vi "addNullElement.vi"(7 "Name":string, 8 "error in (no error)":errorcluster, 10 "Replace? (false)":bool, 11 "tBSONDocument in":refnum<class "tBSONDocument.lvclass">) -> (0 "error out":errorcluster, 3 "tBSONDocument out":refnum<class "tBSONDocument.lvclass">)   [LabVIEW 2013, in "BSON.lvlib" / "tBSONDocument.lvclass"]
doc: "Adds an Null element to a BSON document."
uses:
  tBSONDocument.lvclass
  BSONElements/tBSONNull/tBSONNull.lvclass
  tBSONElement/tBSONElement.lvclass
  tBSONElement/setName.vi
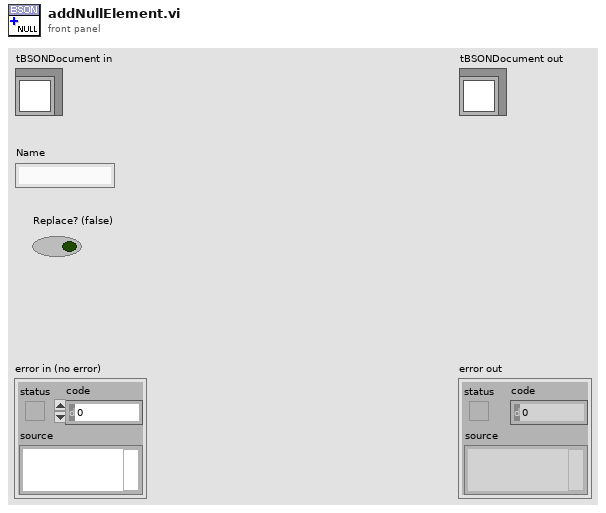
[diagram p1: front panel]
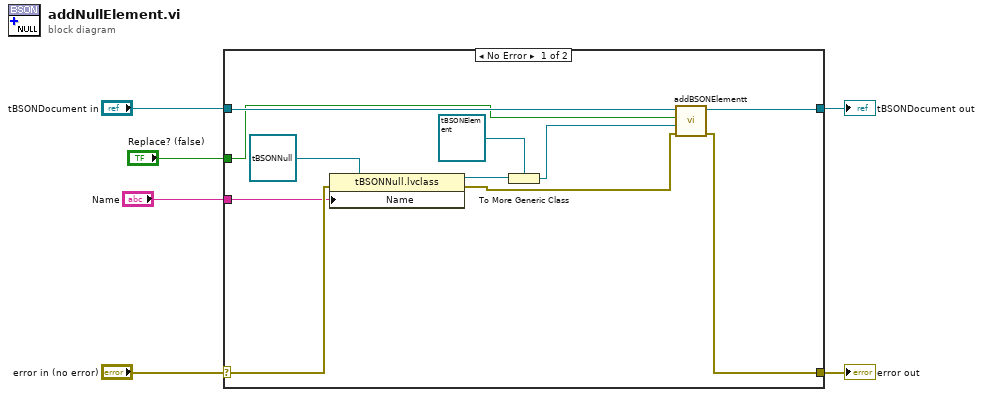
[diagram p0: block diagram]
diagram:
  n1 = case shown="No Error" "error in (no error)" {
    selector: "error in (no error)" -> [w16 w19]
    tunnel: [w9 w19] -> w5
    tunnel: [w8 w18] -> w3
    tunnel: "tBSONDocument in" -> [w14 w18]
    tunnel: "Name" -> [w15 _]
    tunnel: "Replace? (false)" -> [w7 _]
    frame No Error {
      n2 = property class="tBSONNull.lvclass"(reference=refnum<class "tBSONNull.lvclass"> refnum ("BSON.lvlib:tBSONNull.lvclass"), error in=w16, "Name"=w15) -> (reference out=w13:refnum<class "tBSONNull.lvclass">, error out=w10:errorcluster)
      n3 = To More Generic Class(target class=refnum<class "tBSONElement.lvclass"> refnum ("BSON.lvlib:tBSONElement.lvclass"), reference=w13) -> (generic class reference=w11:refnum<class "tBSONElement.lvclass">)
      n4 = call "addBSONElementt.vi"("error in (no error)"=w10, "Element"=w11, "Replace? (false)"=w7, "tBSONDocument in"=w14) -> ("error out"=w9:errorcluster, "tBSONDocument out"=w8:refnum<class "tBSONDocument.lvclass">)  [unwired: 6 in]
    }
    frame Error {
    }
  }
  "error out" <- w5
  "tBSONDocument out" <- w3
